vi "Tag Viewer.vi"() -> ()   [LabVIEW 2017]
uses:
  <vilib>/Skyline/Tag/Wrapper/Wrapper_class/NI Skyline Tag.lvclass/NI Skyline Tag.ctl
  <vilib>/Skyline/Tag/Wrapper/Wrapper_class/Read Tag Path.vi
  <vilib>/Skyline/Tag/Wrapper/Wrapper AMQP_class/Query Tags AMQP.vi
  <vilib>/Skyline/Tag/Wrapper/Wrapper_class/Read Tag (DBL).vi
  <vilib>/Skyline/Tag/Wrapper/Wrapper_class/Read Tag (I32).vi
  <vilib>/Skyline/Tag/Wrapper/Wrapper_class/Read Tag (String).vi
  <vilib>/Skyline/Tag/Wrapper/Wrapper_class/NI Skyline Tag.lvclass
  <vilib>/Skyline/Tag/Wrapper/Wrapper AMQP_class/NI Skyline Tag AMQP.lvclass
panel:
  out "Number of tags":i32
  out "Tags":string[][](table)
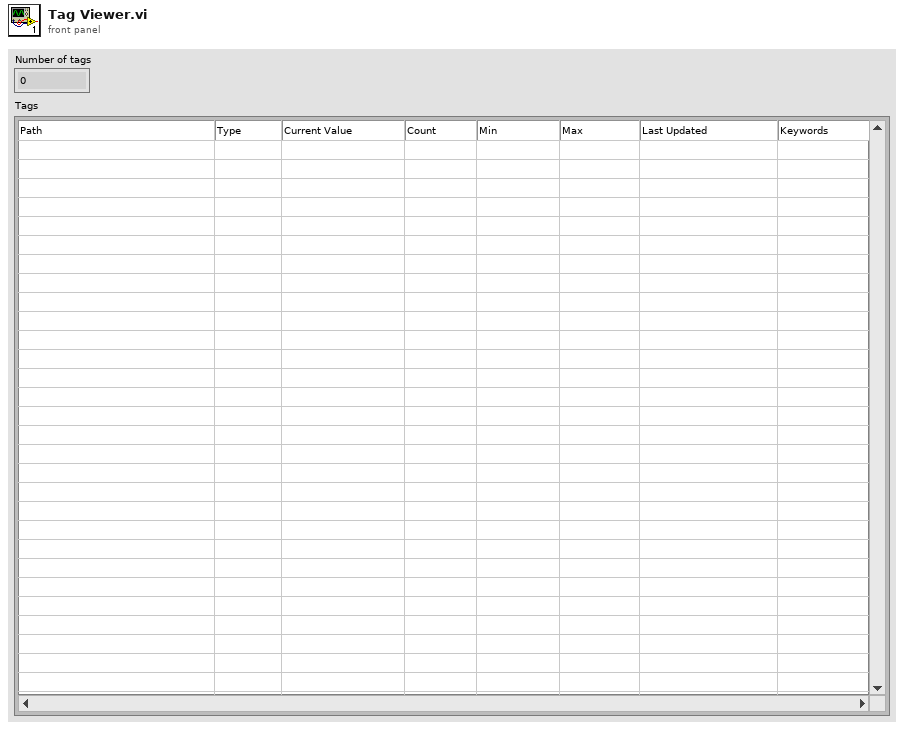
[diagram p1: front panel]
types:
  T1 = typedef "NI Skyline Tag.lvlib/DataType.ctl" = enum32{"Double", "Integer", "String"}
  T2 = typedef "NI Skyline Tag.lvlib/Aggregates Double.ctl" = cluster{"Count":i32, "Max":dbl, "Min":dbl, "Mean":dbl}
  T3 = typedef "NI Skyline Tag.lvlib/Aggregates Int.ctl" = cluster{"Count":i32, "Max":i32, "Min":i32, "Mean":dbl}
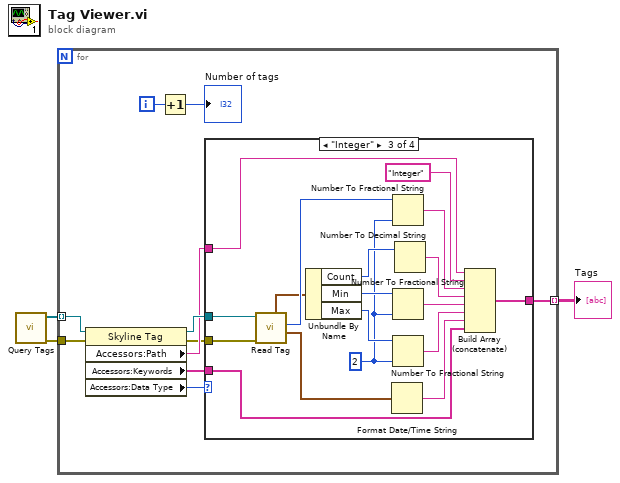
[diagram p0: block diagram]
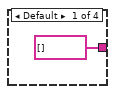
[diagram p2: hidden frame]
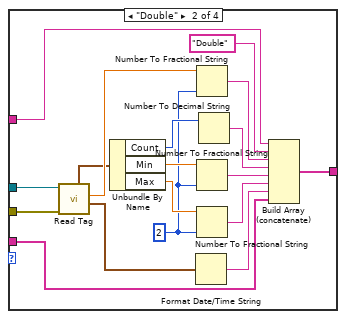
[diagram p3: hidden frame]
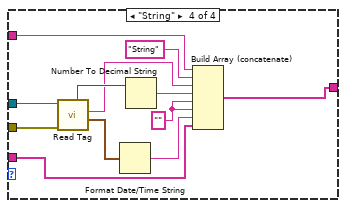
[diagram p4: hidden frame]
diagram:
  n1 = call-poly <vilib>:"Query Tags.vi"() -> ("error out"=w1:errorcluster, "tags"=w3:refnum<class "NI Skyline Tag.lvclass">[])  [unwired: 10 in]
  n2 = for {
    tunnel: w3 -> [w13] mode=indexing
    tunnel: [w10] -> w2 mode=indexing
    tunnel: w1 -> [w8]
    i -> [w5]
    n3 = property class="Skyline Tag"(reference=w13, error in=w8) -> (reference out=w12:refnum<class "NI Skyline Tag.lvclass">, error out=w7:errorcluster, "Accessors:Path"=w11:string, "Accessors:Keywords"=w9:string[], "Accessors:Data Type"=w4:T1)
    n4 = Increment(x=w5) -> (x+1=→"Number of tags":i32)
    n5 = case shown="\"Integer\"" w4 {
      tunnel: w12 -> [_ w32 w50 w62]
      tunnel: w11 -> [_ w26 w44 w60]
      tunnel: [string[] [] w21 w39 w58] -> w10
      tunnel: w9 -> [_ w18 w36 w56]
      tunnel: w7 -> [_ w17 w35 w55]
      frame Default {
      }
      frame "Double" {
        w20 = i16 2 ("precision (6)")
        n6 = call-poly <vilib>:"Read Tag.vi"("error in (no error)"=w17, "tag in"=w32) -> ("time stamp"=w30:timestamp, "value"=w31:dbl, "Aggregate Values"=w16:T2)  [unwired: 5 in, 2 out]
        n7 = Unbundle By Name(w16) -> ("Count"=w29:i32, "Min"=w28:dbl, "Max"=w27:dbl)
        n8 = Format Date/Time String(seconds (now)=w30) -> (date/time string=w19:string)  [unwired: 2 in]
        n9 = Number To Fractional String(number=w31, precision (6)=w20) -> (F-format string=w25:string)  [unwired: 2 in]
        n10 = Number To Fractional String(number=w28, precision (6)=w20) -> (F-format string=w23:string)  [unwired: 2 in]
        n11 = Number To Fractional String(number=w27, precision (6)=w20) -> (F-format string=w22:string)  [unwired: 2 in]
        n12 = Number To Decimal String(number=w29) -> (decimal integer string=w24:string)  [unwired: 1 in]
        n13 = Build Array (concatenate)(w26, "Double" ("element"), w25, w24, w23, w22, w19, w18) -> (w21:string[])
      }
      frame "Integer" {
        w38 = i16 2 ("precision (6)")
        n14 = call-poly <vilib>:"Read Tag.vi"("error in (no error)"=w35, "tag in"=w50) -> ("time stamp"=w48:timestamp, "value"=w49:i32, "Aggregate Values"=w34:T3)  [unwired: 5 in, 2 out]
        n15 = Unbundle By Name(w34) -> ("Count"=w47:i32, "Min"=w46:i32, "Max"=w45:i32)
        n16 = Format Date/Time String(seconds (now)=w48) -> (date/time string=w37:string)  [unwired: 2 in]
        n17 = Number To Fractional String(number=w49, precision (6)=w38) -> (F-format string=w43:string)  [unwired: 2 in]
        n18 = Number To Fractional String(number=w46, precision (6)=w38) -> (F-format string=w41:string)  [unwired: 2 in]
        n19 = Number To Fractional String(number=w45, precision (6)=w38) -> (F-format string=w40:string)  [unwired: 2 in]
        n20 = Number To Decimal String(number=w47) -> (decimal integer string=w42:string)  [unwired: 1 in]
        n21 = Build Array (concatenate)(w44, "Integer" ("element"), w43, w42, w41, w40, w37, w36) -> (w39:string[])
      }
      frame "String" {
        w52 = "" ("element")
        n22 = call-poly <vilib>:"Read Tag.vi"("error in (no error)"=w55, "tag in"=w62) -> ("time stamp"=w61:timestamp, "value"=w53:string, "count"=w54:i32)  [unwired: 5 in, 2 out]
        n23 = Format Date/Time String(seconds (now)=w61) -> (date/time string=w57:string)  [unwired: 2 in]
        n24 = Number To Decimal String(number=w54) -> (decimal integer string=w59:string)  [unwired: 1 in]
        n25 = Build Array (concatenate)(w60, "String" ("element"), w53, w59, w52, w52, w57, w56) -> (w58:string[])
      }
    }
  }
  "Tags" <- w2
